vi "Coordenadas de rescate.vi"(0 "VISA resource name":refnum<visa-resource-name>, 1 "X1":i32, 2 "Y1":i32, 3 "X2":i32, 4 "Y2":i32, 5 "error in (no error)":errorcluster, 6 "X3":i32, 7 "Y3":i32, 8 "X4":i32, 9 "Y4":i32, 10 "X5":i32, 11 "Y5":i32) -> (14 "VISA resource name out":refnum<visa-resource-name>, 19 "error out":errorcluster)   [LabVIEW 2021]
panel:
  in  "Y6":i32
  in  "X6":i32
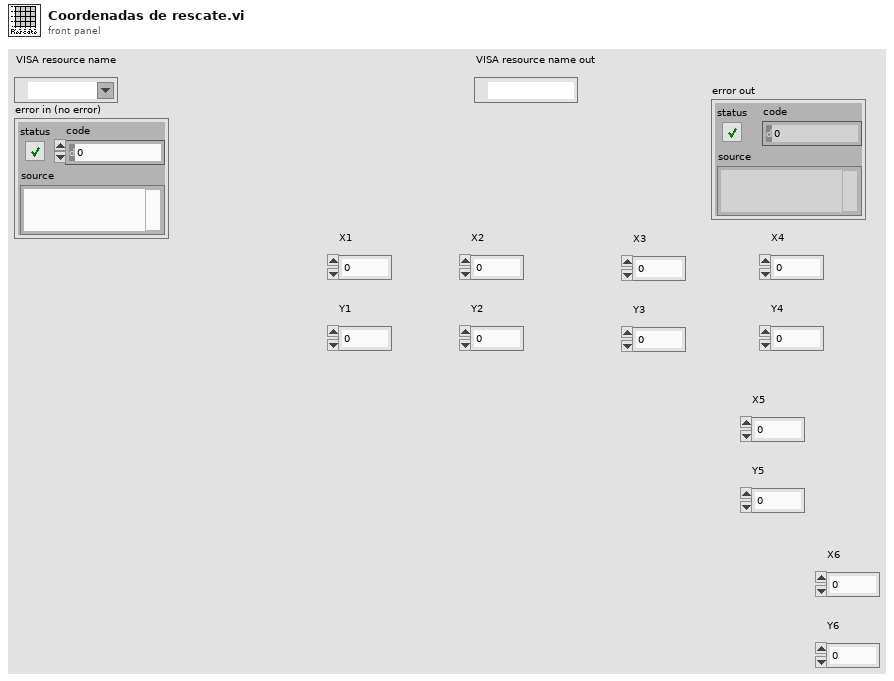
[diagram p1: front panel]
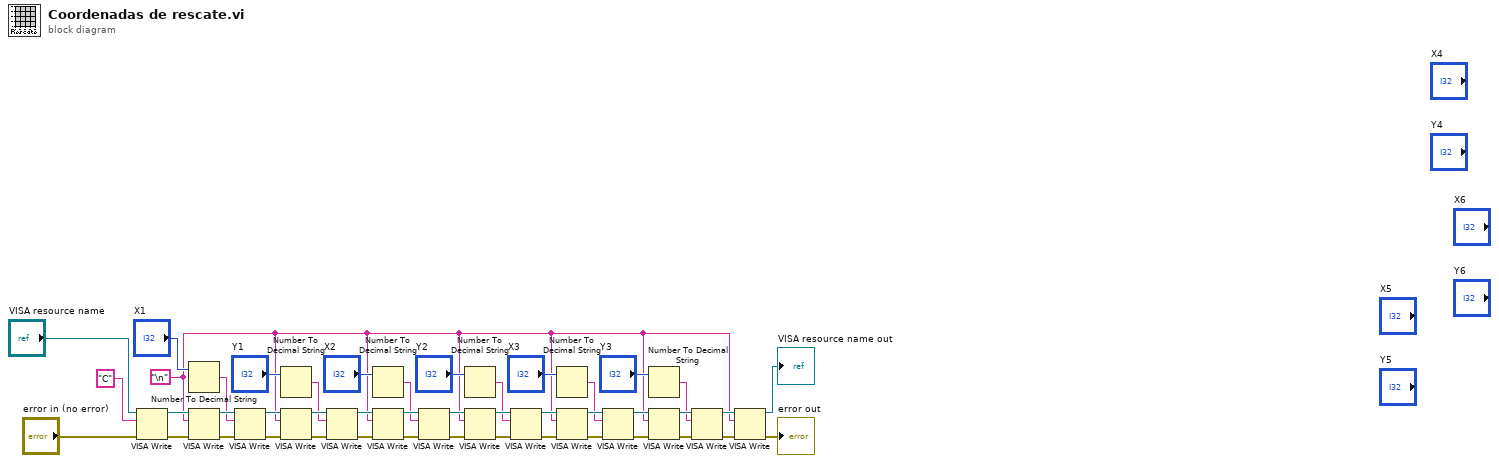
[diagram p0: block diagram]
diagram:
  w3 = "\n"
  n1 = VISA Write(VISA resource name="VISA resource name", write buffer="C", error in (no error)="error in (no error)") -> (VISA resource name out=w42:refnum<visa-resource-name>, error out=w43:errorcluster)  [unwired: 1 out]
  n2 = Number To Decimal String(number="X1") -> (decimal integer string=w28:string)  [unwired: 1 in]
  n3 = VISA Write(VISA resource name=w42, write buffer=w3, error in (no error)=w43) -> (VISA resource name out=w40:refnum<visa-resource-name>, error out=w41:errorcluster)  [unwired: 1 out]
  n4 = VISA Write(VISA resource name=w40, write buffer=w28, error in (no error)=w41) -> (VISA resource name out=w38:refnum<visa-resource-name>, error out=w39:errorcluster)  [unwired: 1 out]
  n5 = Number To Decimal String(number="Y1") -> (decimal integer string=w27:string)  [unwired: 1 in]
  n6 = VISA Write(VISA resource name=w38, write buffer=w3, error in (no error)=w39) -> (VISA resource name out=w37:refnum<visa-resource-name>, error out=w36:errorcluster)  [unwired: 1 out]
  n7 = VISA Write(VISA resource name=w37, write buffer=w27, error in (no error)=w36) -> (VISA resource name out=w35:refnum<visa-resource-name>, error out=w34:errorcluster)  [unwired: 1 out]
  n8 = Number To Decimal String(number="X2") -> (decimal integer string=w17:string)  [unwired: 1 in]
  n9 = VISA Write(VISA resource name=w35, write buffer=w3, error in (no error)=w34) -> (VISA resource name out=w25:refnum<visa-resource-name>, error out=w26:errorcluster)  [unwired: 1 out]
  n10 = VISA Write(VISA resource name=w25, write buffer=w17, error in (no error)=w26) -> (VISA resource name out=w23:refnum<visa-resource-name>, error out=w24:errorcluster)  [unwired: 1 out]
  n11 = Number To Decimal String(number="Y2") -> (decimal integer string=w16:string)  [unwired: 1 in]
  n12 = VISA Write(VISA resource name=w23, write buffer=w3, error in (no error)=w24) -> (VISA resource name out=w21:refnum<visa-resource-name>, error out=w22:errorcluster)  [unwired: 1 out]
  n13 = VISA Write(VISA resource name=w21, write buffer=w16, error in (no error)=w22) -> (VISA resource name out=w19:refnum<visa-resource-name>, error out=w20:errorcluster)  [unwired: 1 out]
  n14 = Number To Decimal String(number="X3") -> (decimal integer string=w6:string)  [unwired: 1 in]
  n15 = VISA Write(VISA resource name=w19, write buffer=w3, error in (no error)=w20) -> (VISA resource name out=w14:refnum<visa-resource-name>, error out=w15:errorcluster)  [unwired: 1 out]
  n16 = VISA Write(VISA resource name=w14, write buffer=w6, error in (no error)=w15) -> (VISA resource name out=w12:refnum<visa-resource-name>, error out=w13:errorcluster)  [unwired: 1 out]
  n17 = Number To Decimal String(number="Y3") -> (decimal integer string=w4:string)  [unwired: 1 in]
  n18 = VISA Write(VISA resource name=w12, write buffer=w3, error in (no error)=w13) -> (VISA resource name out=w10:refnum<visa-resource-name>, error out=w11:errorcluster)  [unwired: 1 out]
  n19 = VISA Write(VISA resource name=w10, write buffer=w4, error in (no error)=w11) -> (VISA resource name out=w8:refnum<visa-resource-name>, error out=w9:errorcluster)  [unwired: 1 out]
  n20 = VISA Write(VISA resource name=w8, write buffer=w3, error in (no error)=w9) -> (VISA resource name out=→"VISA resource name out":refnum<visa-resource-name>, error out=→"error out":errorcluster)  [unwired: 1 out]
